vi "getparam.vi"(8 "error in (no error)":errorcluster, 11 "Input":string="34,45,89") -> (0 "error out":errorcluster, 3 "Output":string)   [LabVIEW 2014]
uses:
  <userlib>/Nanonis Prog Interface V5/Scan/Piezos/Piezo Calibration Range Get.vi
  <userlib>/Nanonis Prog Interface V5/Nanonis Prog Interface.lvlib
panel:
  out "size(s)":i32=3
  # "."
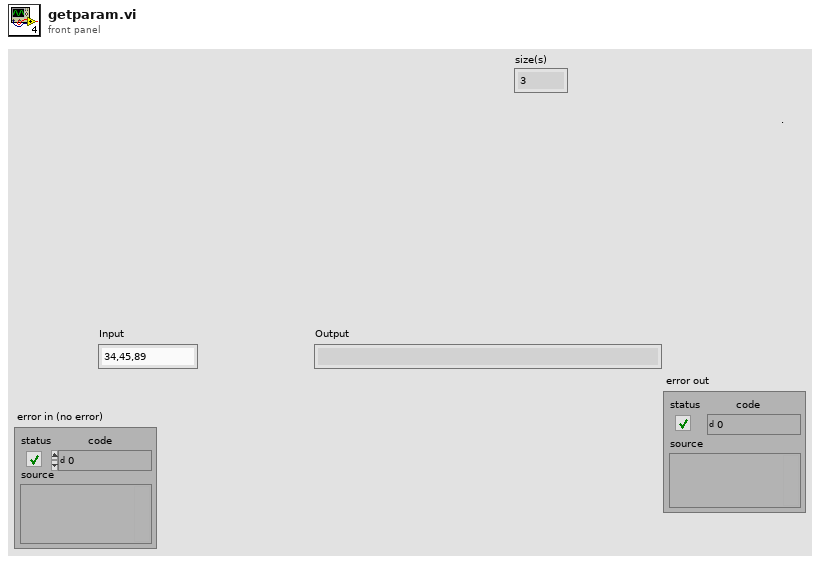
[diagram p1: front panel]
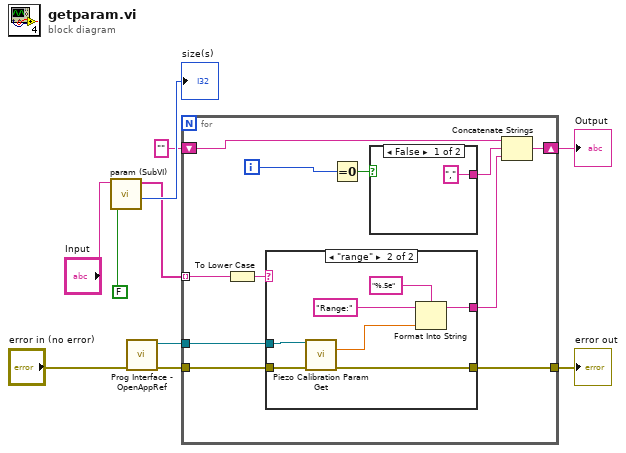
[diagram p0: block diagram]
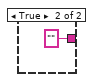
[diagram p2: hidden frame]
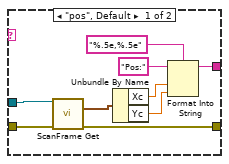
[diagram p3: hidden frame]
diagram:
  n1 = call <userlib>:"param (SubVI).vi"("Numeric"=FALSE, "Input"="Input") -> ("num"=→"size(s)":i32, "Array"=w6:string[])  [unwired: 7 in, 1 out]
  n2 = call <userlib>:"Prog Interface - OpenAppRef.vi"("Error in (no error)"="error in (no error)") -> ("Error out"=w3:errorcluster, "Application reference"=w5:refnum<vi>)  [unwired: 5 in]
  n3 = for {
    tunnel: w6 -> [w21] mode=indexing
    tunnel: w5 -> [w20]
    shift-right: [w16] -> w1
    shift-left: "" -> [w19]
    tunnel: w3 -> [w15]
    tunnel: [w14] -> w2
    i -> [w11]
    n4 = To Lower Case(string=w21) -> (all lower case string=w13:string)
    n5 = case shown="\"range\"" w13 {
      tunnel: w20 -> [w32 w39]
      tunnel: [w25 w35] -> w17
      tunnel: w15 -> [w31 w34]
      tunnel: [w24 w33] -> w14
      frame "pos", Default {
        n6 = call <userlib>:"ScanFrame Get.vi"("Application ref in"=w32, "error in (no error)"=w31) -> ("Center coordinates (m)"=w30:cluster{"Xc":sgl, "Yc":sgl}, "error out"=w24:errorcluster)  [unwired: 9 in, 3 out]
        n7 = Unbundle By Name(w30) -> ("Xc"=w27:sgl, "Yc"=w26:sgl)
        n8 = Format Into String(format string="%.5e,%.5e", initial string="Pos:", w27, w26) -> (resulting string=w25:string)  [unwired: 1 in, 1 out]
      }
      frame "range" {
        n9 = call-poly <userlib>:"Piezo Calibration Param Get.vi"("Application ref in"=w39, "error in (no error)"=w34) -> ("Range X (m)"=w37:sgl, "error out"=w33:errorcluster)  [unwired: 9 in, 3 out]
        n10 = Format Into String(format string="%.5e", initial string="Range:", w37) -> (resulting string=w35:string)  [unwired: 1 in, 1 out]
      }
    }
    n11 = Equal To 0?(x=w11) -> (x = 0?=w12:bool)
    n12 = case shown="False" w12 {
      tunnel: ["," ("string") "" ("string")] -> w18
      frame False {
      }
      frame True {
      }
    }
    n13 = Concatenate Strings(w19, w18, w17) -> (w16:string)
  }
  "Output" <- w1
  "error out" <- w2
